vi "Config PressureDisplay.vi"(8 "error in (no error)":errorcluster, 11 "Configuration in":refnum<class "Configuration.lvclass">) -> (0 "error out":errorcluster, 3 "Configuration out":refnum<class "Configuration.lvclass">)   [LabVIEW 2016, in "Hardware.lvlib" / "VacuumLine.lvlib" / "VacuumLines Configuration.lvclass"]
uses:
  <userlib>/Common Components/Hardware/Abstract System/VacuumLine/VacuumLines Configuration/VacuumLines Configuration.lvclass
  <userlib>/Configuration Dialog Actor/Configuration.lvclass
  <userlib>/Common Components/Hardware/Abstract System/VacuumLine/VacuumLines/Gauge Param.ctl
  C:/Program Files (x86)/National Instruments/LabVIEW 2016/user.lib/Configuration Dialog Actor/Configuration.lvclass
  <userlib>/Common Components/Hardware/Abstract System/VacuumLine/VacuumLines Configuration/VacuumLines Configuration.lvclass/VacuumLines Configuration.ctl
  <userlib>/Common Components/Hardware/Abstract System/VacuumLine/VacuumLines/VacuumLines.lvclass
panel:
  in  "PressureDisplay Setup":T1[](array[typedef]) {"Threshold" format="%#.1e"}
  in  "Revert":bool
  in  "Apply":bool
  # "Label"
  # "Gauge Controller"
  # "Channel"
  # "Threshold"
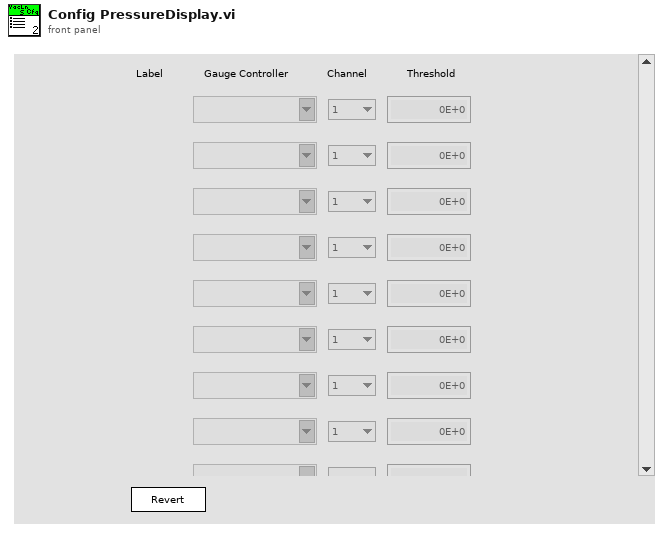
[diagram p1: front panel]
types:
  T1 = typedef "Hardware.lvlib/VacuumLine.lvlib/VacuumLines.lvclass/Gauge Param.ctl" = cluster{"label":string, "Gauge Controller":string, "Channel":enum16{"1", "2", "3", "4", "5", "6", "7", "8"}, "Threshold":dbl}
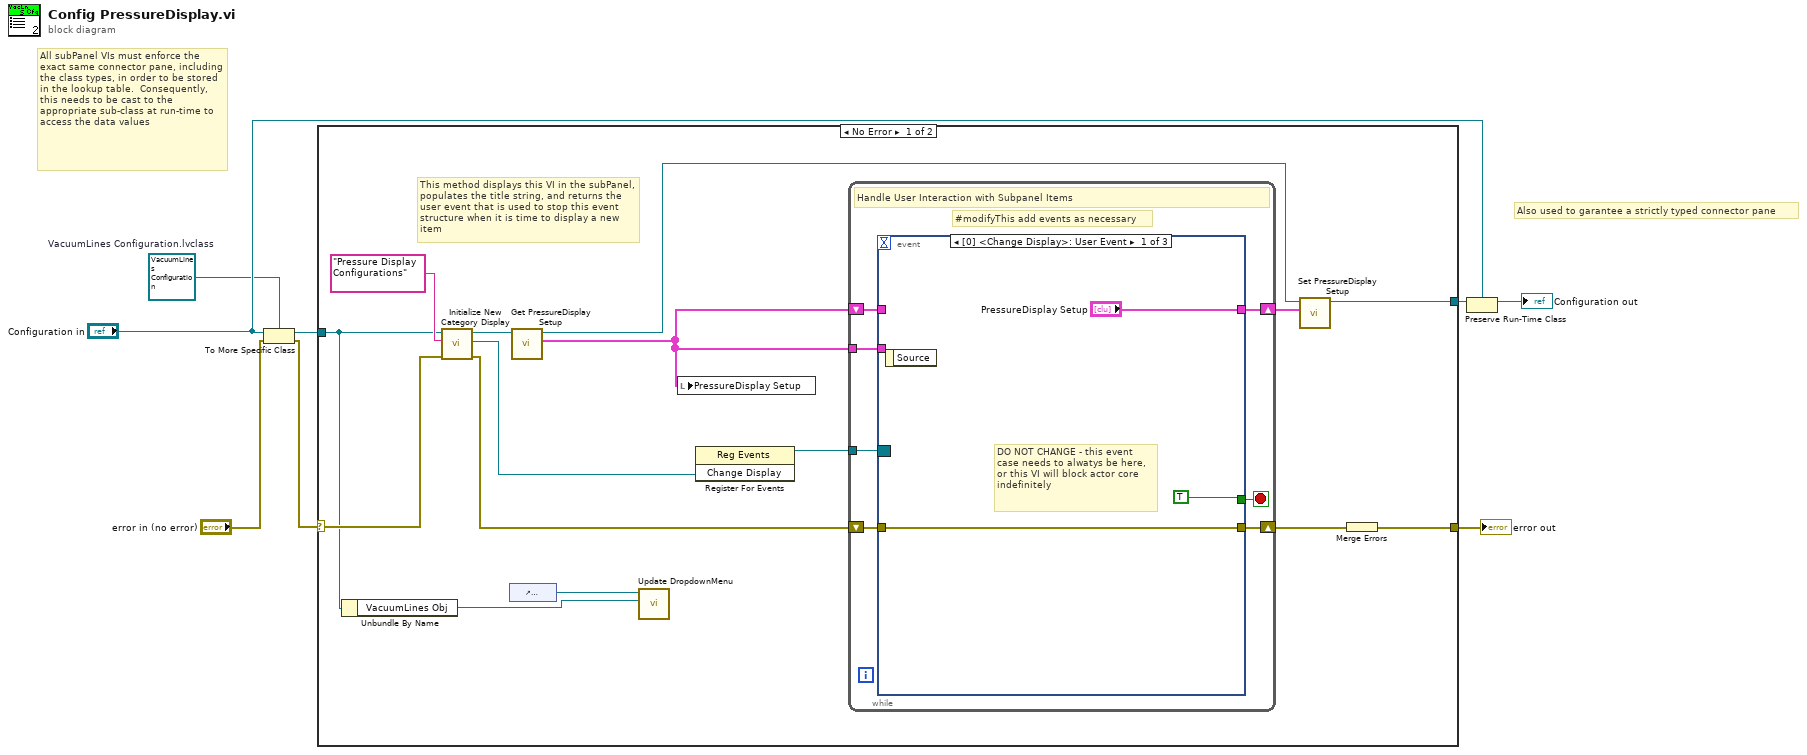
[diagram p0: block diagram]
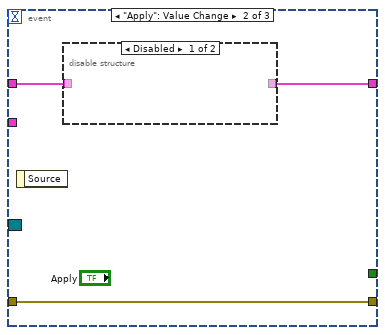
[diagram p2: hidden frame]
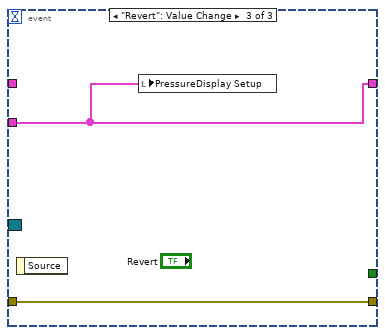
[diagram p4: hidden frame]
diagram:
  w2 = refnum<class "VacuumLines Configuration.lvclass"> refnum  # VacuumLines Configuration.lvclass
  # "Also used to garantee a strictly typed connector pane"
  # "All subPanel VIs must enforce the exact same connector pane, including the class types, in order to be stored in the lookup table.  Consequently, this needs to be cast to the appropriate sub-class at run-time to access the data values"
  n1 = To More Specific Class(target class=w2, reference="Configuration in", error in="error in (no error)") -> (specific class reference=w6:refnum<class "VacuumLines Configuration.lvclass">, error out=w1:errorcluster)
  n2 = case shown="No Error" w1 {
    selector: w1 -> [w17 w40]
    tunnel: w6 -> [w12 w41]
    tunnel: [w14 w41] -> w8
    tunnel: [w23 w40] -> w7
    frame No Error {
      # "This method displays this VI in the subPanel, populates the title string, and returns the user event that is used to stop this event structure when it is time to display a new item"
      n3 = Unbundle By Name(w12) -> ("VacuumLines Obj"=w11:refnum<class "VacuumLines.lvclass">)
      n4 = call <userlib>:"Initialize New Category Display.vi"("error in (no error)"=w17, "Name to Display"="Pressure Display Configurations", "Configuration in"=w12) -> ("error out"=w18:errorcluster, "Change Display"=w21:refnum<user-event>, "Configuration Out"=w16:refnum<class "VacuumLines Configuration.lvclass">)  [unwired: 6 in]
      n5 = control-ref of="PressureDisplay Setup"() -> (w9:refnum<vi>)
      n6 = call <userlib>:"Get PressureDisplay Setup.vi"("VacuumLines Configuration in"=w16) -> ("PressureDisplay Setup"=w13:T1[], "VacuumLines Configuration out"=w15:refnum<class "VacuumLines Configuration.lvclass">)  [unwired: 8 in, 1 out]
      n7 = call <userlib>:"Update DropdownMenu.vi"("VacuumLines Obj"=w11, "Ref of Array"=w9) -> ()  [unwired: 10 in]
      n8 = local write "PressureDisplay Setup"(w13) -> ()
      n9 = register-events(w21) -> (reference out=w20:refnum<event-registration>)  [unwired: 2 in, 1 out]
      n10 = while {
        tunnel: w20 -> [w29]
        shift-right: [w28] -> w19
        shift-left: w18 -> [w27]
        shift-right: [w25] -> w10
        shift-left: w13 -> [w26]
        tunnel: w13 -> [w24]
        stop <- w30 stop-if-true
        # "#modifyThis add events as necessary"
        # "Handle User Interaction with Subpanel Items"
        n11 = event shown="[0] <Change Display>: User Event" {
          selector: w29 -> [_ _ _]
          dyn-events: _ -> [_ _ _]
          timeout: _ -> [_ _ _]
          tunnel: [TRUE _ _] -> w30
          tunnel: [w33 w36 w39] -> w28
          tunnel: w27 -> [w33 w36 w39]
          tunnel: w26 -> [_ w34 _]
          tunnel: ["PressureDisplay Setup" w35 w38] -> w25
          tunnel: w24 -> [_ _ w38]
          event User Event {
            # "DO NOT CHANGE - this event case needs to alwatys be here, or this VI will block actor core indefinitely"
            n12 = event-data() -> ()  [unwired: 1 in, 1 out]
          }
          event "Apply": Value Change {
            n13 = event-data() -> ()  [unwired: 1 in, 1 out]
            n14 = disable-structure shown="Disabled" {
              disable-tunnel: [_ w37] -> w35
              disable-tunnel: w34 -> [_ w37]
              frame Disabled {
              }
              frame Enabled {
              }
            }
          }
          event "Revert": Value Change {
            n15 = event-data() -> ()  [unwired: 1 in, 1 out]
            n16 = local write "PressureDisplay Setup"(w38) -> ()
          }
        }
      }
      n17 = call <userlib>:"Set PressureDisplay Setup.vi"("PressureDisplay Setup"=w10, "VacuumLines Configuration in"=w15) -> ("VacuumLines Configuration out"=w14:refnum<class "VacuumLines Configuration.lvclass">)  [unwired: 8 in, 1 out]
      n18 = Merge Errors(w19) -> (w23:errorcluster)
    }
    frame Error {
    }
  }
  "error out" <- w7
  n19 = Preserve Run-Time Class(object in=w8, 2:"Configuration in") -> (object out=→"Configuration out":refnum<class "Configuration.lvclass">)  [unwired: 1 in, 1 out]
